vi "FTW-Time-Elapse.vi"(10 "End Time":u32, 11 "Initial Time":u32) -> (2 "Elapsed sec":dbl format="%08.3fsec", 3 "Elapsed msec":u32 format="%06dmsec")   [LabVIEW 2014]
panel:
  # "Inputs"
  # "Outputs"
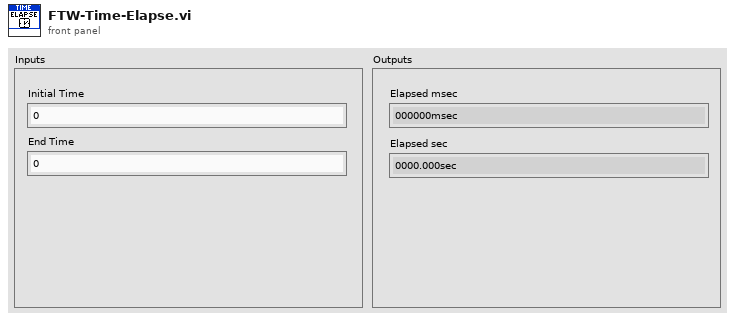
[diagram p1: front panel]
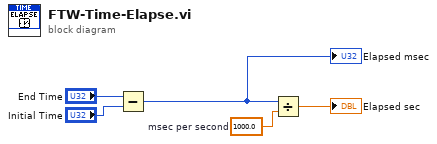
[diagram p0: block diagram]
diagram:
  w5 = 1000.0  # msec per second
  n1 = Subtract(x="End Time", y="Initial Time") -> (x-y=w2:u32)
  "Elapsed msec" <- w2
  n2 = Divide(x=w2, y=w5) -> (x/y=→"Elapsed sec":dbl)
